vi "Sub Initialize.vi"(6 "Controller name":string, 8 "error in (no error)":errorcluster, 11 "Instrument Recorder in":refnum<class "Pulse Recorder Actor.lvclass">) -> (0 "error out":errorcluster, 2 "Initialize Result":refnum<class "Acquired Result.lvclass">, 3 "Instrument Recorder out":refnum<class "Pulse Recorder Actor.lvclass">)   [LabVIEW 2021, in "Pulse Recorder Actor.lvclass"]
uses:
  Pulse Recorder Actor.lvclass
  Pulse Recorder Actor.lvclass/Pulse Recorder Actor.ctl
  Instrument Actor/Instrument Actor.lvclass
  NHMFL_Core/Libraries/Instruments/Results/Acquired Result/Acquired Result.lvclass
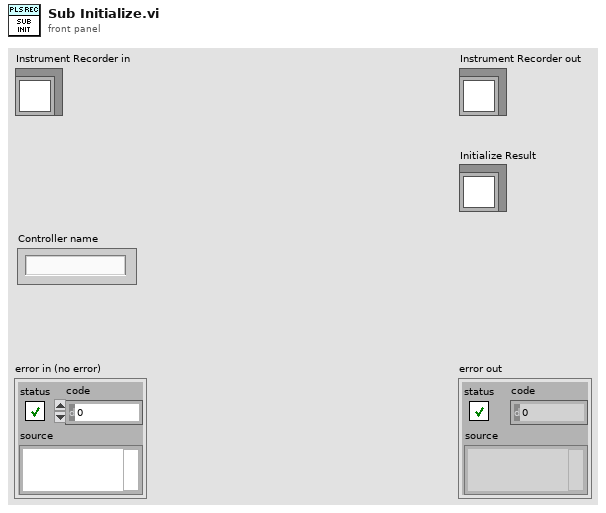
[diagram p1: front panel]
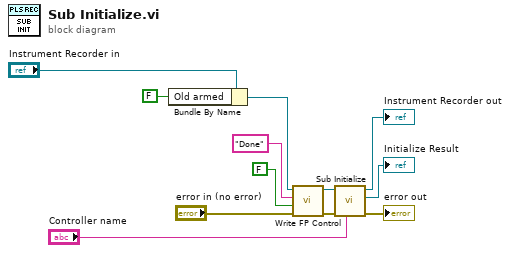
[diagram p0: block diagram]
diagram:
  n1 = Bundle By Name(cluster="Instrument Recorder in", "Old armed"=FALSE ("Armed")) -> (w4:refnum<class "Pulse Recorder Actor.lvclass">)
  n2 = call-dynamic "Write FP Control.vi"("error in (no error)"="error in (no error)", "Control Value"=FALSE, "Control Name"="Done", "Measure Object in"=w4) -> ("error out"=w5:errorcluster, "Measure Object out"=w3:refnum<class "Pulse Recorder Actor.lvclass">)  [unwired: 6 in]
  n3 = call-parent "Sub Initialize.vi"("Controller name"="Controller name", "error in (no error)"=w5, "Instrument Recorder in"=w3) -> ("error out"=→"error out":errorcluster, "Initialize Result"=→"Initialize Result":refnum<class "Acquired Result.lvclass">, "Instrument Recorder out"=→"Instrument Recorder out":refnum<class "Pulse Recorder Actor.lvclass">)  [unwired: 6 in]
